vi "Create JSON Response Message.vi"(10 "Data":string) -> (2 "Message":string)   [LabVIEW 2024, in "Sift Client.lvlib"]
uses:
  Sift Client.lvlib
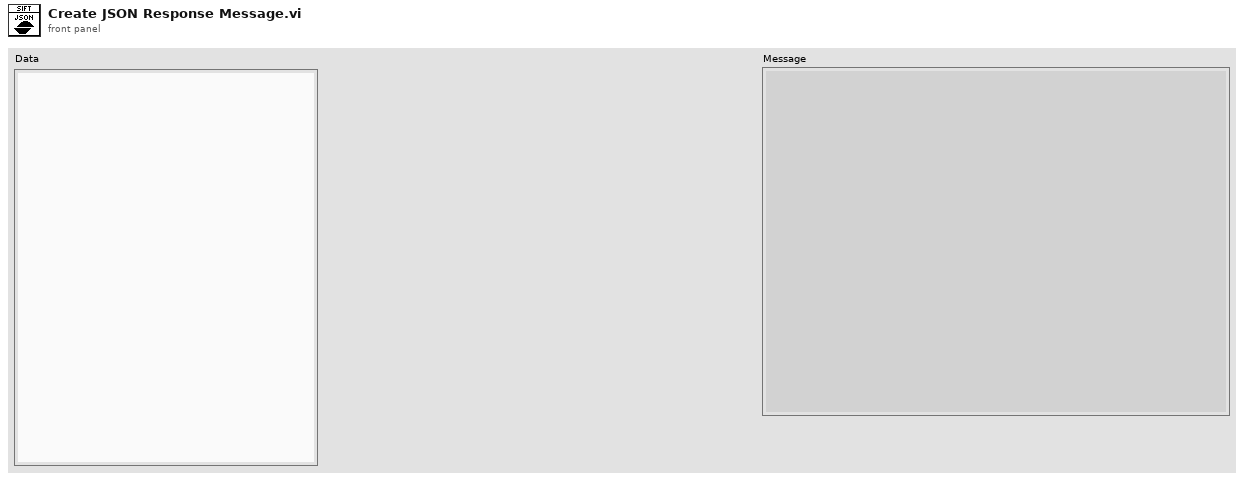
[diagram p1: front panel]
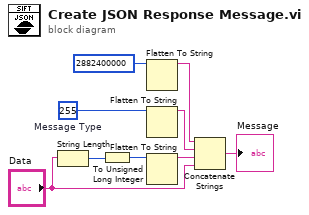
[diagram p0: block diagram]
diagram:
  w9 = u8 255  # Message Type
  n1 = String Length(string="Data") -> (length=w2:i32)
  n2 = To Unsigned Long Integer(number=w2) -> (unsigned 32bit integer=w1:u32)
  n3 = Flatten To String(anything=u32 2882400000) -> (data string=w3:string)  [unwired: 3 in, 2 out]
  n4 = Flatten To String(anything=w9) -> (data string=w8:string)  [unwired: 3 in, 2 out]
  n5 = Flatten To String(anything=w1) -> (data string=w7:string)  [unwired: 3 in, 2 out]
  n6 = Concatenate Strings(w3, w8, w7, "Data") -> (→"Message":string)
